vi "LD2018_ブロック崩し_ブロック配置.vi"(4 "Yオフセット":i32, 5 "Y":i32, 6 "Xオフセット":i32, 7 "X":i32, 9 "Scrn-BALL位置":T1 caption="Position", 10 "ブロック配列入力":bool[][](array[boolean]), 11 "ブッロクReference":refnum<vi>[][](array[refnum])) -> (2 "ブロック配列出力":bool[][](array[boolean]), 3 "ブッロクReference出力":refnum<vi>[][](array[refnum]))   [LabVIEW 2016]
uses:
  <vilib>/Utility/miscctls.llb/LVPositionTypeDef.ctl
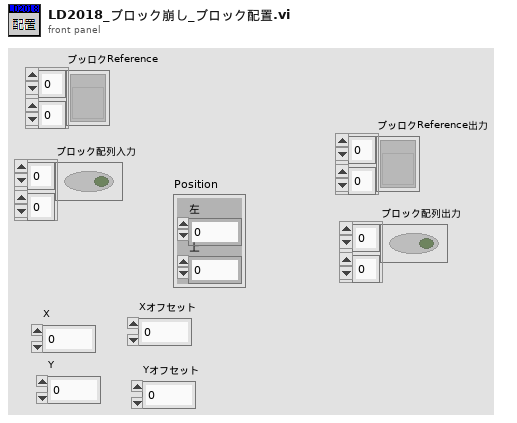
[diagram p1: front panel]
types:
  T1 = typedef "LVPositionTypeDef.ctl" = cluster{"Left":i32, "Top":i32}
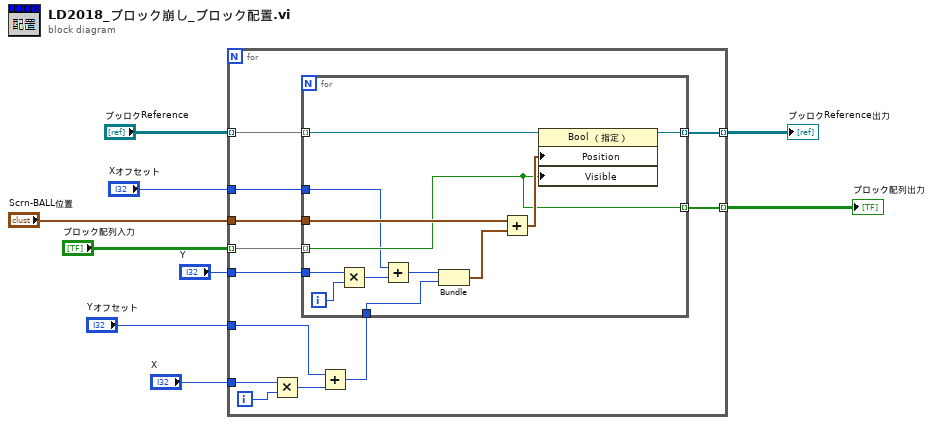
[diagram p0: block diagram]
diagram:
  n1 = for "Forループ" {
    tunnel: "ブッロクReference" -> [w21] mode=indexing
    tunnel: "Scrn-BALL位置" -> [w20]
    tunnel: [w16] -> w2 mode=indexing
    tunnel: [w15] -> w3 mode=indexing
    tunnel: "ブロック配列入力" -> [w14] mode=indexing
    tunnel: "X" -> [w13]
    tunnel: "Y" -> [w12]
    tunnel: "Xオフセット" -> [w11]
    tunnel: "Yオフセット" -> [w10]
    i -> [w19]
    n2 = Multiply(x=w13, y=w19) -> (x*y=w18:i32)
    n3 = Add(x=w10, y=w18) -> (x+y=w17:i32)
    n4 = for "Forループ" {
      tunnel: w21 -> [w33] mode=indexing
      tunnel: w20 -> [w28]
      tunnel: w17 -> [w29]
      tunnel: [w25] -> w16 mode=indexing
      tunnel: [w24] -> w15 mode=indexing
      tunnel: w14 -> [w24] mode=indexing
      tunnel: w12 -> [w23]
      tunnel: w11 -> [w22]
      i -> [w32]
      n5 = Multiply(x=w23, y=w32) -> (x*y=w31:i32)
      n6 = Add(x=w22, y=w31) -> (x+y=w30:i32)
      n7 = Bundle(w30, w29) -> (w26:cluster{i32, i32})  [unwired: 1 in]
      n8 = Add(x=w28, y=w26) -> (x+y=w27:T1)
      n9 = property class="Bool （指定）"(reference=w33, "Position"=w27, "Visible"=w24) -> (reference out=w25:refnum<vi>)  [unwired: 1 in, 1 out]
    }
  }
  "ブロック配列出力" <- w3
  "ブッロクReference出力" <- w2
